vi "CvrtRow2Data.vi"(8 "error in (no error)":errorcluster, 9 "Item Names":string[](array[string]), 10 "ge_DAQManDefinitions":T1, 11 "MeasType":T2) -> (0 "error out":errorcluster, 3 "Channel out":refnum<class "Channel.lvclass">)   [LabVIEW 2018]
uses:
  Custom Ctrls/ge_MeasType.ctl
  Common/Controls/DAQMan Definitions.ctl
  Classes/Measurements/Class Channel/Channel.lvclass
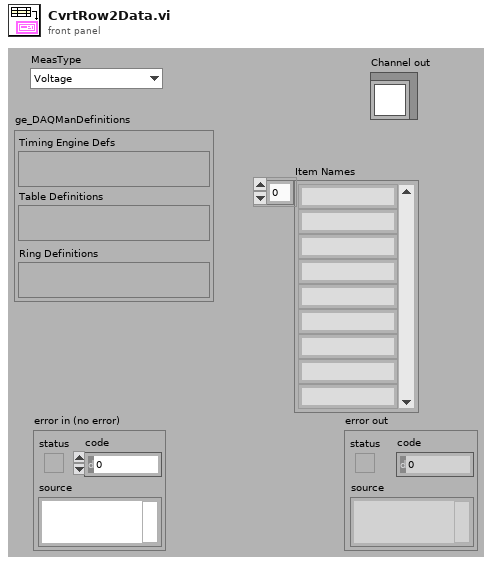
[diagram p1: front panel]
types:
  T1 = typedef "DAQMan Definitions.ctl" = cluster{"Timing Engine Defs":variant, "Table Definitions":variant, "Ring Definitions":variant}
  T2 = typedef "ge_MeasType.ctl" = enum16{"Voltage", "Frequency", "Tachometer", "Dynamic", "Thermocouple", "RTD", "Strain", "Current", "Resistance"}
  T3 = typedef "ge_ColDef.ctl" = cluster{"ge_HdrNames":T4, "HdrInfo":T5}
  T4 = typedef "HeaderNames.ctl" = enum16{"Channel", "Device", "Spacer", "Description", "MB", "Range", "Terminal", "Coupling", "Thresh (V)", "Pulse/Rev", "Slope", "Min EU", "Min RPM", "mV/EU", "Iex", "Temp Units", "Type", "CJC Src", "CJC Val", "Ro", "Wire Cfg", "Strain Mode", "Vex", "Bridge Type", "GF", "Gauge Res", "Poisson", "Lead Res", "Init Strain", "GAF", "Scale", "Offset", "Unit (EU)", "dB?", "dB Ref", "Cal Mag", "Cal Units", "Max Temp", "Min Temp", "Max Strain", "Min Strain"}
  T5 = typedef "ge_HdrInfo.ctl" = cluster{"Hdr Width":i32, "Glbl Ctrl":T6}
  T6 = typedef "ge_GlblCtrls.ctl" = enum16{"Str0", "Bool0", "Bool1", "Int0", "Ring0", "Ring1", "Ring2", "Ring3", "Dbl0", "Dbl1", "Dbl2", "Dbl3", "Cal0", "Cal1", "Cal2", "None"}
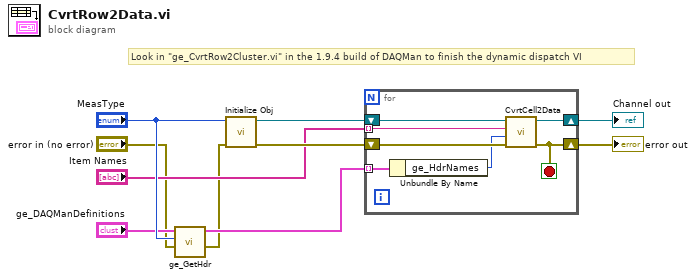
[diagram p0: block diagram]
diagram:
  # "Look in \"ge_CvrtRow2Cluster.vi\" in the 1.9.4 build of DAQMan to finish the dynamic dispatch VI"
  n1 = call "ge_GetHdr.vi"("error in"="error in (no error)", "MeasType"="MeasType", "ge_DAQManDefinitions"="ge_DAQManDefinitions") -> ("error out"=w1:errorcluster, "Table Hdrs"=w8:T3[])  [unwired: 7 in]
  n2 = call "Initialize Obj.vi"("error in (no error)"=w1, "MeasType"="MeasType") -> ("error out"=w9:errorcluster, "Channel out"=w10:refnum<class "Channel.lvclass">)  [unwired: 8 in]
  n3 = for {
    shift-right: [w17] -> w7
    shift-left: w10 -> [w16]
    shift-right: [w11] -> w6
    shift-left: w9 -> [w15]
    tunnel: "Item Names" -> [w14] mode=indexing
    tunnel: w8 -> [w13] mode=indexing
    stop <- w11 stop-if-true
    n4 = Unbundle By Name(w13) -> ("ge_HdrNames"=w12:T4)
    n5 = call-dynamic "CvrtCell2Data.vi"("error in (no error)"=w15, "Header Names"=w12, "Item Name"=w14, "Channel in"=w16) -> ("error out"=w11:errorcluster, "Channel out"=w17:refnum<class "Channel.lvclass">)  [unwired: 6 in]
  }
  "Channel out" <- w7
  "error out" <- w6
